vi "act-5NI - sous-VI.vi"() -> ()   [LabVIEW 2010]
uses:
  act/lv_07/lv_07.lvlib
panel:
  in  "error out":errorcluster caption="err out"
  out "err in":errorcluster
  out "TE":dbl
  in  "T":dbl
  in  "CC":dbl
  out "Qe":dbl
  in  "Pu":dbl
  in  "Qa":dbl
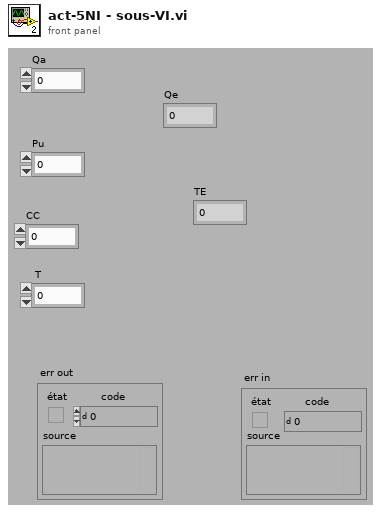
[diagram p1: front panel]
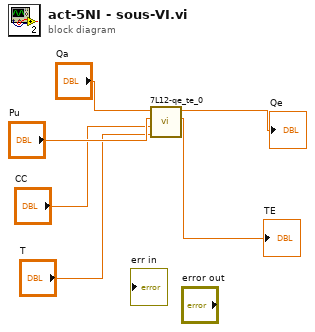
[diagram p0: block diagram]
diagram:
  n1 = call "7L12-qe_te_0.vi"("Cc"="T", "T"="CC", "Pu"="Pu", "Qa"="Qa") -> ("Te (en mois)"=→"TE":dbl, "Qe"=→"Qe":dbl)  [unwired: 5 in, 1 out]
